vi "21_2.vi"() -> ()   [LabVIEW 2020]
uses:
  <userlib>/_OpenG.lib/array/array.llb/Remove Duplicates from 1D Array (String)__ogtk.vi
  <userlib>/_OpenG.lib/array/array.llb/Index 1D Array Elements (String)__ogtk.vi
panel:
  out "spreadsheet string":string
  in  "Switch":bool
  in  "Input":string="tksps nmzblnq pzz gkmdkp fdpp htdps njvzpr lsfn vxbnd qvft rggkbpj nmpt ptq dckbmh bh xxlb pbjp zlpbptr mmphj ddc zxmkkpp jrgrcz xzhmdb mqkf bmcj nmtzlj dxzq lsv bsbz fvqg mklt dlkxsxg nkmj crbt zxcqtf rjbsr hbcgjtx vvqpqgl rnbfzg hxndkq vrntfjx clmk zdslsk ljczhn fkntrq kbkkrlfq bt mrz nhpsk lsc vqjj gpxmf lfd bsllxjtm zdpcb qpjplfl gkcskhp vrbxt mxf ftnhrx fbjbkp sffzz (contains fish, soy)\npzvvt phth fvqg mlftm gpxmf kbkkrlfq nmtzlj dtqq jdnlg dlxp ljczhn zrngn qnlrbn lbxc chjdk fkntrq xxlb pcvh xmgc vkzh pzz sgv xlc xmjr bqtpqsp vrntfjx xxx dlkxsxg xzhmdb vpsd clptg qpjplfl fcrvj nmzblnq cxgmp jqcfq sbr xbdmll jtknrjp fcdtf bbxvmgs mgjdd dckbmh lmxt dxzq ns fdpp pbjp xbtpfxjz fbvdlb mrz ftnhrx fsddds hsmkqgx gkmdkp xxdmj cksrd zgbbl zdslsk zpqbb bgkf rnbfzg bhgzdg ndmjr nhpsk mxf fjndll cfnc pmqmmxs rqpd mqkf snpxpkvj (contains shellfish)\nbh dxzq zbsqdm lxkbkkx lcpcmk xbdmll ttszmr pzvvt jbhhjx qfqnpf dckbmh zgbbl vrbxt rggkbpj dzbxmn bsllxjtm dblf mlftm fvqg htdps ldprd tllqrt sfprzmk zrngn lmxfpn hxndkq gkcskhp bqtpqsp chjdk kzfsztx nkmj tjxxdmq ztlp dlkxsxg vvzf vplt bhgzdg gsshb lmxt bmjx fjndll clmk qbrgtl ndmjr nmtzlj xzhmdb bpzlm kspf gvhrgz ddcrr fdpp tlgbjhs gpxmf xvqmjsc lsc mqkf lsv krrsrp zsbzn bkxnht mgjdd jbtjxtf slbrp kchnq vpsd zdpcb ftnhrx sm mcdsfh xplxv fkntrq gntk tksps sbr vbxdp vtdd lrbpxs dgnrq ktm (contains sesame, eggs, peanuts)\nxlc dlkxsxg jrgrcz lkdrpt rqpd xgzbl fjndll ddcrr xbhsqv pqjgdkl fvqg mxf lxkbkkx kttchg vvzf xxdmj xzhmdb pbjp fcdtf kbkkrlfq bpzlm qlbxr lmxt rggkbpj ptq kzfsztx dgnrq jbhhjx vqjj qnlrbn kckgz cnmm nmtzlj zgbbl lrbpxs ztlp hnlcp zhlgsj bgkf zdpcb xbtpfxjz bsllxjtm krrsrp pzz nhpsk mrz ndmjr zmqvhh xxlb dxzq bqtpqsp zsbzn (contains dairy, sesame)\nqlgb ztlp gvhrgz sfprzmk vcvmq xxlb lmxfpn njrdhq lcpcmk ttszmr qbrgtl tnzvgg hbfmpsg hshl vvqpqgl pzz dckbmh zlpbptr slbrp xgxk dlkxsxg mxf qlbxr bmcj bqtpqsp hsmkqgx ftnhrx qmxfh fvqg lbnr hbcgjtx krrsrp nmpt fxznf zpqbb lmxt vbxdp dtqq dxzq zdslsk nmtzlj mgjdd gpxmf vtdd kttchg rdtkzbf qfqnpf ndmjr zrngn (contains wheat, fish)\nttszmr bqtpqsp qvft nhpsk qfqnpf pcvh dxzq qmxfh cksrd xxlb mcdsfh bhgzdg nklz fcdtf mqkf pkzjrp phth zpqbb xvqmjsc pbjp dlxp fcrvj sfprzmk hnlcp xbtpfxjz hxndkq gkmdkp vxbnd pzz clptg mlftm nmzblnq pmqmmxs cpjsfp gpxmf cfnc xmjr nmpt sbr vvqpqgl fxznf mcrxr hgvszq ftnhrx dlkxsxg vpsd vqjj bsbz pmvs gntk fvqg bt kckgz fzpcbck ddc tjxxdmq vjpcxq nmtzlj mxf lmxt prjcx pzvvt mgjdd (contains fish)\nnjrdhq xxx sffzz cksrd gvhrgz nkmj xvqmjsc mxf dxzq jglfn cxgmp fkntrq vxbnd bkdpdr ddcrr hxndkq jclqn mrz vrntfjx fbjbkp nmpt slbrp mcrxr tnzvgg krrsrp jtknrjp hsmkqgx gpxmf pmqmmxs xxlb pbjp ndmjr xlc sbr gxnxkkh bsd kzfsztx vvzf qmxfh jrmj tksps kchnq dgnrq nmfd mcdsfh zmqvhh bcv qvft gsshb kspf lsfn zxmkkpp pqjgdkl fvqg tlgbjhs hgvszq nmtzlj xbhsqv rggkbpj rqpd xmgc kfghxt tjxxdmq bmcj rjbsr fmfj zhlgsj zsbzn xmjr ktm fcrvj pzvvt vbxdp zpqbb pkzjrp fcdtf ddc crbt kckgz dmrxd pmsjc lmxt nmzblnq phth qpjplfl fsddds vplt bsbz (contains dairy, wheat)\ndlkxsxg vplt nkmj bmjx vvzf rdtkzbf qpjplfl tlgbjhs hsmkqgx dxzq mgjdd bsd mklt xmjr gpxmf xxdmj bkdpdr fbjbkp fvqg ktm crbt mxf nmtzlj vpsd pzz fzpcbck krrsrp zpqbb cvrqg vcvmq xxlb vtdd htdps vvqpqgl lsv clptg kttchg jbtjxtf ljczhn vjpcxq dblf sfprzmk bqtpqsp dgnrq fcdtf dzbxmn pzvvt chjdk jtknrjp rggkbpj vf ptq ddcrr lsc njvzpr jrgrcz gkmdkp nklz lsfn ttszmr jrmj mqkf jglfn jdnlg pmvs dtqq (contains fish, wheat, shellfish)\nbsd jbtjxtf nmtzlj njvzpr dlkxsxg dblf hqvv bkxnht dzjjxr xbtpfxjz fxznf cvrqg qpjplfl kspf fcdtf hbcgjtx mxf lsfn zhlgsj dmrxd lsc lkdrpt nmpt dlxp hshl jclqn fkntrq sffzz lxkbkkx lsv dxzq mcrxr mgjdd bt zxcqtf zgbbl bh rggkbpj pthjxs htdps gpxmf pkzjrp fbjbkp lmxt vbxdp kbkkrlfq pmvs pcvh zdpcb ns (contains peanuts, fish, dairy)\nvrntfjx dxzq zdpcb vbxdp lmxt jbtjxtf zhlgsj xbdmll qlbxr xmjr qpjplfl pqjgdkl gsshb rggkbpj fkntrq mcdsfh ddcrr bt fbvdlb jqcfq bgkf dtqq fmfj ddc bsllxjtm kbkkrlfq cpjsfp jbhhjx qlgb vrbxt fbjbkp gntk zrngn kckgz nmtzlj zlpbptr qvft hnlcp lrbpxs bkxnht dlkxsxg cksrd vqjj sgv dmrxd slbrp rkzkd pthjxs cvrqg fcrvj vtdd kchnq qbrgtl mlftm mxf fdpp zmqvhh jrgrcz pzz kttchg xvqmjsc pcvh ttszmr fvqg pzvvt bmjx gkcskhp gvhrgz (contains eggs, fish)\ncnmm lmxt krrsrp kbkkrlfq fvqg dlkxsxg gpxmf gsshb vbxdp sgv kzfsztx zbsqdm kttchg gvhrgz rkzkd jtknrjp hsmkqgx rjbsr hbcgjtx bsllxjtm dmrxd dzbxmn jglfn vpsd tsnzbdtb vcvmq xxx zlpbptr fbjbkp lbnr dxzq hnlcp mcrxr rggkbpj tllqrt lsc fjndll bbxvmgs tksps bmjx xmjr mlftm nmtzlj (contains eggs, dairy, shellfish)\nqlgb ljczhn tjxxdmq gpxmf mrz kttchg pzz xmjr vvzf ktm zhlgsj zsbzn dckbmh lmxt nmtzlj vcvmq jglfn zxmkkpp fxznf xmgc hgvszq zlpbptr mxf hbfmpsg tsnzbdtb dxzq lkdrpt vbxdp pqjgdkl mlftm nhpsk ptq vjpcxq gsshb cfnc ddcrr kckgz bh kzfsztx tnzvgg fvqg dblf xbdmll vkzh pmqmmxs dlkxsxg vplt nklz xplxv gvhrgz lsfn jclqn lxkbkkx prjcx mklt hsmkqgx vtdd sm (contains sesame, peanuts, fish)\nvrntfjx rjbsr bmcj lxkbkkx pmqmmxs zpqbb zmqvhh cfnc nmtzlj dgnrq qpjplfl fcdtf zsbzn fvqg zrngn vqjj dlkxsxg nmzblnq ldprd qvft fzpcbck xxx cpjsfp xlc lmxt clptg tksps sffzz vvzf mxf rggkbpj gvhrgz jrgrcz nhpsk lmxfpn dzjjxr sgv tjxxdmq pbjp jdnlg tllqrt vxbnd htdps tlgbjhs lfd gpxmf pmsjc jglfn nmpt xbtpfxjz vplt gntk (contains shellfish, peanuts, fish)\nvtdd zdslsk rqpd zdpcb vkzh clptg ldprd jglfn ztlp mxf vrbxt vplt zbsqdm zhlgsj crbt bcv nhpsk jbtjxtf tllqrt xbtpfxjz pzvvt lkdrpt kttchg tlgbjhs vvzf kbkkrlfq fbvdlb sffzz ddcrr rggkbpj dlxp dckbmh gvhrgz bgkf dxzq fvqg hxndkq lbnr slbrp bsd hsmkqgx zpqbb gntk lcpcmk lmxt ptq gxnxkkh nkmj vf xgxk hgvszq ns jdnlg dlkxsxg qmxfh ddc mqkf fkntrq njrdhq gpxmf gkmdkp (contains shellfish, dairy)\ngpxmf qmxfh bh lbnr fvqg lsc xlc rggkbpj fzpcbck fbvdlb njvzpr qlgb gkmdkp xxx nhpsk bcv nmtzlj cpjsfp lmxt rjbsr vvzf tsnzbdtb lbxc ptq xvqmjsc mxf lrbpxs qpjplfl rqpd tjxxdmq ktm qlbxr sfprzmk dlkxsxg xgxk ldprd phth fcdtf dmrxd vtdd zmqvhh nmfd xxlb qvft mlftm bpzlm zlpbptr fjndll vqjj zpqbb kbkkrlfq vf (contains eggs, fish, soy)\ngvhrgz xplxv lsfn mmphj nmpt dzjjxr qnlrbn tjxxdmq slbrp chjdk kchnq ftnhrx xxdmj gkcskhp rkzkd mcdsfh nmtzlj tlgbjhs hgvszq bqtpqsp bmjx ndmjr hxndkq xxx dzbxmn htdps ldprd xmjr jclqn rggkbpj mxf qbrgtl pbjp zxcqtf zlpbptr xlc hbfmpsg hshl lrbpxs lsv vplt vf mklt gpxmf tsnzbdtb sm bcv lmxt bhgzdg pmvs fbvdlb clptg sbr pmsjc tllqrt fkntrq kckgz fsddds lsc xbhsqv zmqvhh bpzlm qvft fbjbkp lcpcmk vrntfjx fvqg mqkf vxbnd dlkxsxg rdtkzbf ljczhn ptq fcrvj vpsd (contains soy)\nrkzkd qfqnpf zrngn ftnhrx lmxt lkdrpt qnlrbn fvqg ljczhn hxndkq vrntfjx xplxv lxkbkkx bqtpqsp tksps mxf mgjdd pmqmmxs crbt zgbbl dzjjxr fsddds pzvvt lrbpxs lcpcmk pthjxs qlgb gpxmf zmqvhh rggkbpj dgnrq nhpsk lsv bkdpdr fdpp vkzh vvzf dxzq dlkxsxg sbr vtdd nmzblnq bt zdslsk tjxxdmq xxlb njrdhq xbdmll clmk pcvh mcdsfh (contains shellfish, dairy)\nhsmkqgx crbt lbnr jtknrjp bt nhpsk htdps hgvszq xplxv zxcqtf cnmm jbhhjx gkmdkp nmtzlj xzhmdb ddcrr gkcskhp pbjp fjndll xbhsqv lmxfpn dgnrq kttchg dxzq mcrxr sffzz vbxdp dmrxd hbcgjtx fvqg qlgb xbdmll mxf dtqq rggkbpj bgkf gpxmf cpjsfp vpsd lmxt qpjplfl fxznf ftnhrx jglfn (contains peanuts, wheat, sesame)\ndmrxd fmfj jglfn mqkf zdslsk pmqmmxs xmgc lxkbkkx ndmjr dblf kckgz crbt zmqvhh dzjjxr pkzjrp nmtzlj mgjdd fvqg cpjsfp sm vxbnd kzfsztx sffzz fbvdlb zhlgsj gsshb fjndll hshl rjbsr lsv jqcfq jbtjxtf bkdpdr htdps bsd mrz kttchg kbkkrlfq xzhmdb bhgzdg fkntrq lmxfpn qnlrbn bkxnht njrdhq mklt kchnq cvrqg mcdsfh nmfd xxlb lbnr bh pzz dxzq vvqpqgl fsddds mxf jrmj dlxp lmxt tjxxdmq gpxmf ddc vrbxt hbfmpsg lbxc pzvvt qlbxr sbr hnlcp rnbfzg ttszmr fbjbkp fzpcbck dlkxsxg vkzh lsfn rdtkzbf gkcskhp fdpp (contains shellfish, peanuts, dairy)\nsgv bpzlm vvqpqgl rkzkd dzbxmn phth zsbzn tllqrt bh cpjsfp lmxfpn dlkxsxg mgjdd fbvdlb xzhmdb zbsqdm nhpsk zrngn slbrp zdslsk qnlrbn zmqvhh xxx lxkbkkx pqjgdkl cvrqg jglfn vpsd lsc dxzq hsmkqgx mxf zdpcb gntk xbdmll dgnrq xxdmj dckbmh ldprd rqpd bqtpqsp fvqg gpxmf rggkbpj xbhsqv bcv qlgb gsshb nklz lbxc sffzz lmxt ftnhrx kfghxt nmzblnq kttchg bmcj cnmm snpxpkvj bgkf pmsjc zxcqtf bhgzdg jdnlg zgbbl fsddds ztlp fkntrq (contains wheat, eggs)\nbbxvmgs dlkxsxg bsbz cksrd htdps jrmj fvqg lkdrpt bqtpqsp hshl tnzvgg zxcqtf mklt zsbzn cfnc ns clptg zhlgsj hnlcp jtknrjp tksps vrntfjx fbjbkp gxnxkkh lmxt sffzz rggkbpj sfprzmk bkdpdr xmgc rjbsr lcpcmk vjpcxq nmpt kzfsztx qmxfh nkmj xgzbl jqcfq bh fmfj dblf mxf gpxmf sbr sm gkmdkp nklz vcvmq zdslsk dxzq xbdmll pmvs mrz xlc xxlb lbnr fjndll dzbxmn mqkf xzhmdb nmzblnq zdpcb nmfd lsv qlgb snpxpkvj kchnq qfqnpf lsfn mmphj pkzjrp vbxdp (contains fish)\nvqjj vtdd nmzblnq lbxc zxcqtf xplxv zdpcb lbnr qvft xbtpfxjz bmjx dlkxsxg zmqvhh pzz xxdmj nkmj vvqpqgl bsd tllqrt bpzlm lrbpxs dtqq fvqg lmxfpn lkdrpt fbvdlb vcvmq cnmm dckbmh pmqmmxs tksps njrdhq clptg rggkbpj gpxmf ztlp chjdk tsnzbdtb sgv htdps xmjr kckgz cxgmp dmrxd dblf vpsd rqpd rdtkzbf nmtzlj sm vrntfjx bhgzdg lmxt dxzq ktm cpjsfp ttszmr fdpp kfghxt (contains soy)\nmmphj vvzf fjndll zxcqtf gsshb crbt dtqq cfnc bkdpdr qlbxr fcdtf mxf lcpcmk zdpcb lrbpxs hnlcp zmqvhh snpxpkvj vtdd qpjplfl rggkbpj vrbxt nmfd pzz dlxp jrgrcz vpsd xzhmdb bmjx lkdrpt kzfsztx bqtpqsp jbhhjx pcvh fkntrq chjdk xlc jglfn fsddds tnzvgg mrz ktm gpxmf hbcgjtx lmxfpn jbtjxtf dxzq fvqg zgbbl dlkxsxg ddcrr sgv zxmkkpp kbkkrlfq hxndkq clmk pmqmmxs rdtkzbf mlftm lmxt sffzz tjxxdmq jqcfq xgzbl (contains peanuts)\nqlgb rggkbpj zgbbl lmxt bgkf nmtzlj crbt pcvh clptg hnlcp fzpcbck mqkf kzfsztx hbfmpsg zmqvhh zdpcb pqjgdkl ptq mmphj pmvs vplt xbhsqv mcdsfh rnbfzg sfprzmk cfnc zhlgsj fvqg jbhhjx lfd ztlp lcpcmk lxkbkkx cvrqg njvzpr hbcgjtx ktm mxf xbtpfxjz zlpbptr vbxdp ljczhn nmpt fcdtf tnzvgg qlbxr gpxmf hgvszq xgzbl xzhmdb jrgrcz bbxvmgs mgjdd nklz cnmm bmjx bpzlm dmrxd dckbmh kckgz vqjj lbxc dlxp hshl nkmj fxznf fkntrq clmk bsbz xxdmj vvqpqgl vxbnd chjdk pzvvt dlkxsxg vjpcxq (contains dairy, peanuts)\nqvft zmqvhh gpxmf dlxp zdpcb tlgbjhs fmfj pzz ns bhgzdg vxbnd phth clmk vkzh clptg rggkbpj xmgc lrbpxs dckbmh bmjx fjndll mmphj fcdtf cxgmp lfd vvzf ftnhrx ljczhn lmxt njrdhq dtqq bkxnht zdslsk lsv bsd mlftm bqtpqsp ndmjr mcdsfh kttchg cpjsfp hqvv fbvdlb pmqmmxs sbr tnzvgg kbkkrlfq lkdrpt xlc nmtzlj xvqmjsc fbjbkp ldprd fzpcbck cfnc fkntrq mxf rdtkzbf pmsjc xxx nhpsk jglfn zxmkkpp nmpt hshl xmjr dlkxsxg fvqg zpqbb fdpp vpsd pmvs (contains shellfish, peanuts, fish)\nlbxc tksps mxf ddcrr nmtzlj fdpp zhlgsj xbdmll xlc xvqmjsc vxbnd fxznf clptg pzvvt crbt jbtjxtf rjbsr ddc lmxfpn jclqn mcdsfh xxlb nklz jrgrcz dlkxsxg bqtpqsp zrngn dgnrq clmk mklt ttszmr nmzblnq xzhmdb fkntrq zdslsk xmgc dblf ftnhrx kspf rggkbpj hshl lmxt fvqg dmrxd qvft dzjjxr lxkbkkx nmfd xgxk nhpsk gpxmf vjpcxq (contains soy, sesame, fish)\nnkmj xplxv fvqg jglfn cxgmp zpqbb lsc tllqrt jclqn fxznf lmxt rggkbpj dlkxsxg pcvh xmgc vxbnd vvzf fsddds lmxfpn slbrp hxndkq gpxmf dmrxd snpxpkvj tsnzbdtb gntk phth bqtpqsp cksrd nmtzlj mklt lxkbkkx tnzvgg clptg gvhrgz mqkf rkzkd mrz hshl pthjxs bhgzdg bkdpdr sfprzmk mxf bbxvmgs (contains soy, shellfish)\nclptg tllqrt xbtpfxjz mrz clmk ktm bmjx jclqn xgxk gpxmf nmzblnq lmxt bgkf kzfsztx jrgrcz fkntrq prjcx qbrgtl sffzz kckgz pmqmmxs zgbbl mxf xxlb tlgbjhs cvrqg rjbsr rggkbpj dxzq pmvs xmgc xplxv fsddds fxznf ddc fmfj qlgb xlc lfd hgvszq zmqvhh zhlgsj fzpcbck bhgzdg krrsrp gxnxkkh cksrd lxkbkkx chjdk vrntfjx bsd gkmdkp dblf bsllxjtm nmtzlj vplt mgjdd jglfn njrdhq qfqnpf nmfd sgv vf crbt dlkxsxg (contains wheat, sesame)\ncnmm bbxvmgs nklz prjcx bmcj xxdmj cksrd pmvs vcvmq nmfd tllqrt dckbmh nmzblnq pkzjrp gxnxkkh vbxdp bh lmxt jrgrcz zhlgsj gpxmf rnbfzg ddcrr fcrvj qlgb pmsjc mgjdd zpqbb mxf vrbxt zdslsk dzjjxr qfqnpf vpsd sffzz mklt xbdmll hbcgjtx bt xplxv jglfn kzfsztx dlkxsxg fvqg htdps mcrxr dxzq ldprd nmtzlj vvqpqgl hnlcp kspf bpzlm qnlrbn (contains sesame, soy, fish)\nnjrdhq fzpcbck zsbzn xlc nklz clmk dzbxmn phth nmtzlj dxzq fcdtf chjdk bh slbrp kttchg vkzh bsd gpxmf kchnq lfd bbxvmgs cxgmp bgkf pbjp dlkxsxg xzhmdb hqvv rnbfzg kzfsztx sgv hgvszq zdslsk bkdpdr fsddds pzvvt bmcj sbr mxf ddcrr vbxdp cvrqg mcrxr ldprd ljczhn sffzz pkzjrp jclqn zmqvhh xgxk rggkbpj vvqpqgl cnmm kbkkrlfq xbtpfxjz hxndkq ftnhrx crbt vcvmq nhpsk gsshb bmjx xxlb dckbmh ns lsfn bkxnht bpzlm kfghxt xbhsqv bsllxjtm krrsrp qfqnpf tlgbjhs jbtjxtf tksps hbcgjtx vqjj xvqmjsc tsnzbdtb lrbpxs zhlgsj fjndll bqtpqsp bhgzdg ttszmr hsmkqgx jbhhjx hshl lsc mqkf lmxt jdnlg mgjdd xxx pmvs (contains shellfish, wheat)"
  in  "Input Test":string="mxmxvkd kfcds sqjhc nhms (contains dairy, fish)\ntrh fvjkl sbzzf mxmxvkd (contains dairy)\nsqjhc fvjkl (contains soy)\nsqjhc mxmxvkd sbzzf (contains fish)"
  # "lmxt,rggkbpj,mxf,gpxmf,nmtzlj,dlkxsxg,fvqg,dxzq"
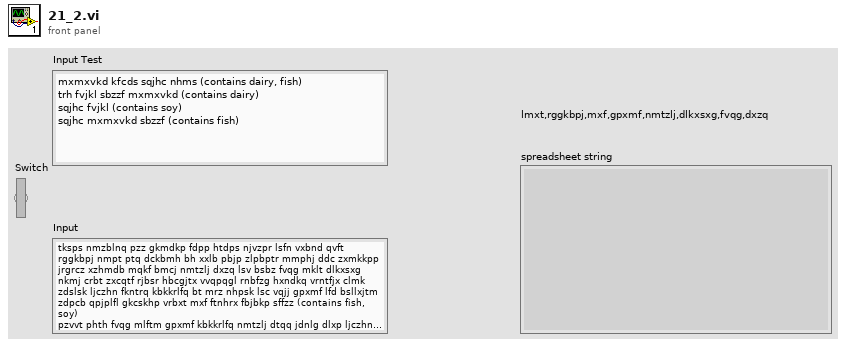
[diagram p1: front panel]
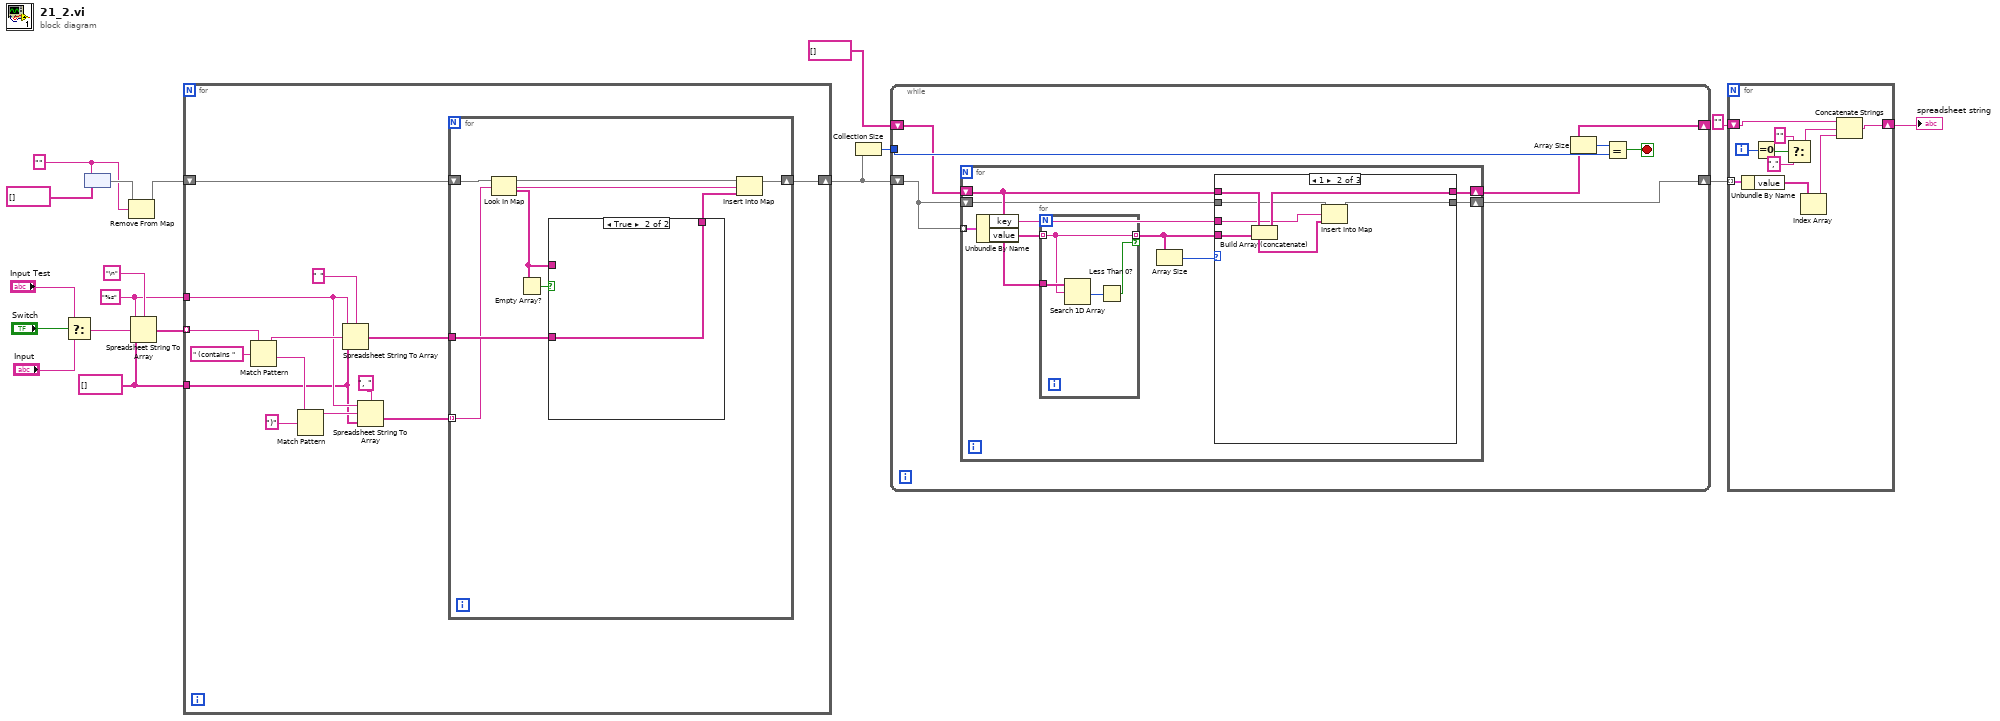
[diagram p0: block diagram]
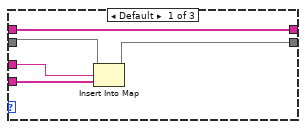
[diagram p2: hidden frame]
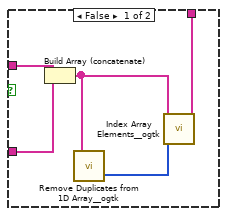
[diagram p4: hidden frame]
diagram:
  w7 = ""
  w10 = string[] []
  w11 = "%s"
  n1 = Select(t="Input Test", s="Switch", f="Input") -> (s? t:f=w15:string)
  n2 = node(w7, string[] []) -> (w9:map{string, string[]})
  n3 = Remove From Map(10:w7, 11:w9) -> (3:w8:map{string, string[]})  [unwired: 2 out]
  n4 = Spreadsheet String To Array(delimiter (Tab)="\n", format string=w11, spreadsheet string=w15, array type (2D Dbl)=w10) -> (array=w13:string[])
  n5 = for {
    tunnel: w13 -> [w32] mode=indexing
    shift-right: [w21] -> w6
    shift-left: w8 -> [w22]
    tunnel: w11 -> [w24]
    tunnel: w10 -> [w23]
    n6 = Match Pattern(string=w32, regular expression=" (contains ") -> (before substring=w30:string, after substring=w28:string)  [unwired: 1 in, 2 out]
    n7 = Match Pattern(string=w28, regular expression=")") -> (before substring=w26:string)  [unwired: 1 in, 3 out]
    n8 = Spreadsheet String To Array(delimiter (Tab)=" ", format string=w24, spreadsheet string=w30, array type (2D Dbl)=w23) -> (array=w19:string[])
    n9 = Spreadsheet String To Array(delimiter (Tab)=", ", format string=w24, spreadsheet string=w26, array type (2D Dbl)=w23) -> (array=w20:string[])
    n10 = for {
      shift-right: [w38] -> w21
      shift-left: w22 -> [w39]
      tunnel: w19 -> [w37]
      tunnel: w20 -> [w35] mode=indexing
      n11 = Look In Map(map=w39, key=w35) -> (value=w34:string[])  [unwired: 1 in, 1 out]
      n12 = Empty Array?(array=w34) -> (empty?=w33:bool)
      n13 = case shown="True" w33 {
        tunnel: w37 -> [w43 w45]
        tunnel: [w41 w45] -> w36
        tunnel: w34 -> [w40 _]
        frame False {
          n14 = Build Array (concatenate)(w40, w43) -> (w42:string[])
          n15 = call-poly <userlib>:"Remove Duplicates from 1D Array__ogtk.vi"("Input Array"=w42) -> ("indices of removed elements"=w44:i32[])  [unwired: 1 out]
          n16 = call-poly <userlib>:"Index Array Elements__ogtk.vi"("indices"=w44, "array"=w42) -> ("elements"=w41:string[])  [unwired: 9 in]
        }
        frame True {
        }
      }
      n17 = Insert Into Map(map in=w39, key=w35, value=w36) -> (map out=w38:map{string, string[]})  [unwired: 2 out]
    }
  }
  n18 = Collection Size(1:w6) -> (0:w4:i32)
  n19 = while {
    shift-right: [w46] -> w3
    shift-left: w6 -> [w47]
    shift-right: [w48] -> _
    shift-left: string[] [] -> [w49]
    tunnel: w4 -> [w51]
    stop <- w50 stop-if-true
    n20 = for {
      tunnel: w47 -> [w61] mode=indexing
      shift-right: [w56] -> w48
      shift-left: w49 -> [w58]
      shift-right: [w54] -> w46
      shift-left: w47 -> [w55]
      n21 = Unbundle By Name(w61) -> ("key"=w53:string, "value"=w60:string[])
      n22 = for {
        tunnel: w60 -> [w77] mode=indexing
        tunnel: w58 -> [w78]
        tunnel: [w77] -> w57 mode=indexing if=w75
        n23 = Search 1D Array(1D array=w78, element=w77) -> (index of element=w76:i32)  [unwired: 1 in]
        n24 = Less Than 0?(x=w76) -> (x < 0?=w75:bool)
      }
      n25 = Array Size(array=w57) -> (size(s)=w59:i32)
      n26 = case shown="1" w59 {
        tunnel: w58 -> [w66 w72 w74]
        tunnel: w57 -> [w63 w68 _]
        tunnel: [w66 w71 w74] -> w56
        tunnel: w55 -> [w64 w70 w73]
        tunnel: [w62 w67 w73] -> w54
        tunnel: w53 -> [w65 w69 _]
        frame Default {
          n27 = Insert Into Map(map in=w64, key=w65, value=w63) -> (map out=w62:map{string, string[]})  [unwired: 2 out]
        }
        frame 1 {
          n28 = Build Array (concatenate)(w72, w68) -> (w71:string[])
          n29 = Insert Into Map(map in=w70, key=w69, value=w68) -> (map out=w67:map{string, string[]})  [unwired: 2 out]
        }
        frame 0 {
        }
      }
    }
    n30 = Array Size(array=w48) -> (size(s)=w52:i32)
    n31 = Equal?(x=w52, y=w51) -> (x = y?=w50:bool)
  }
  n32 = for {
    tunnel: w3 -> [w88] mode=indexing
    shift-right: [w83] -> w1
    shift-left: "" -> [w85]
    i -> [w86]
    n33 = Unbundle By Name(w88) -> ("value"=w87:string[])
    n34 = Equal To 0?(x=w86) -> (x = 0?=w82:bool)
    n35 = Select(t="", s=w82, f=",") -> (s? t:f=w81:string)
    n36 = Index Array(array=w87) -> (element=w84:string)  [unwired: 1 in]
    n37 = Concatenate Strings(w85, w81, w84) -> (w83:string)
  }
  "spreadsheet string" <- w1
